vi "UpdateWeeks (SubVI).vi"(8 "Error In":errorcluster, 11 "DVR In":refnum<data-value>) -> (0 "Error Out":errorcluster, 1 "End Date":timestamp, 2 "Start Date":timestamp, 3 "DVR Out":refnum<data-value>)   [LabVIEW 2017, in "DS_Lib.lvlib" / "SRReportParser.lvlib"]
uses:
  SRReportParser.lvlib
  Modules/Private Controls/Report Data Cluster.ctl
  Modules/Private Controls/Data Raw.ctl
  Modules/Data Operations.lvlib
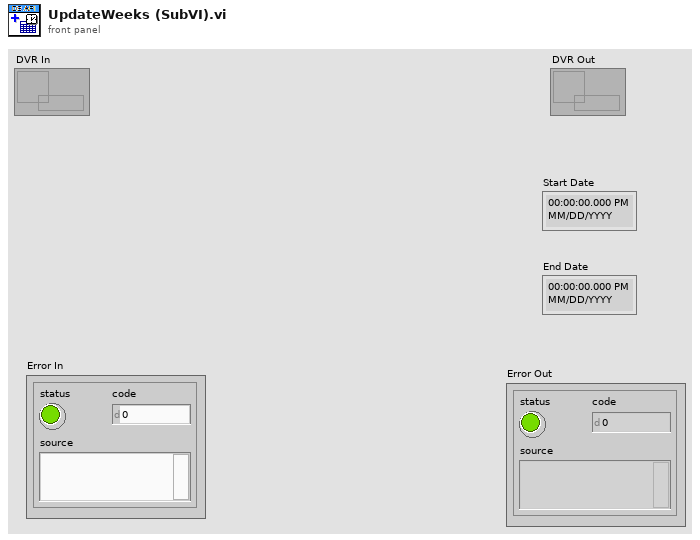
[diagram p1: front panel]
types:
  T1 = typedef "Data Operations.lvlib/Report Data Cluster.ctl" = cluster{"Headers":cluster{"Start Date":timestamp, "End Date":timestamp, "SR Status String":string[], "AE Owner String":string[]}, "Data":T2[]}
  T2 = typedef "Data Operations.lvlib/Data Raw.ctl" = cluster{"SR Number":string, "Status":string, "Summary":string, "AE Owner":string, "AE Group":string, "Contact":string, "SurveyData":cluster{"Resolution Time":dbl, "Total Satisfaction":dbl, "Response Time":dbl, "Courtesy":dbl, "Problem Solved":dbl, "Level of effort":dbl}, "Time Data":cluster{"Last Update Date":timestamp, "Creation Date":timestamp, "Creation week":i16, "Last Update Week":i16, "Creation Year":i16}}
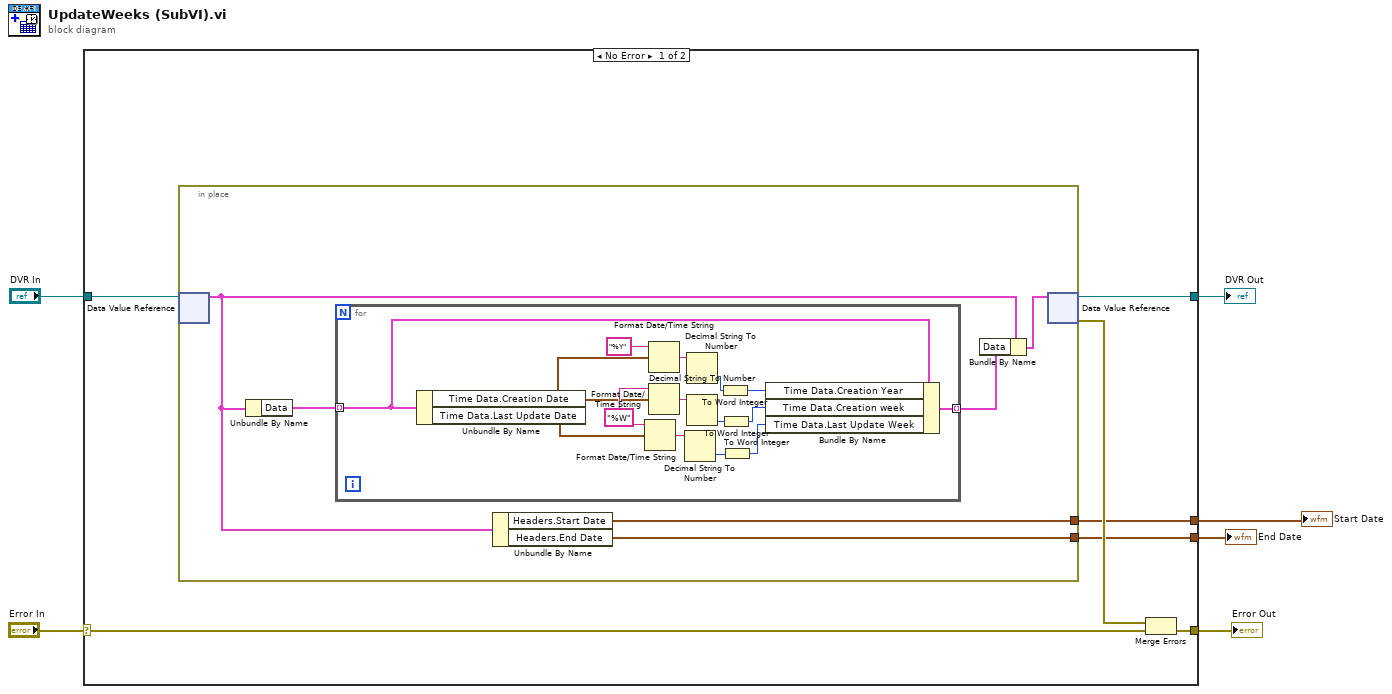
[diagram p0: block diagram]
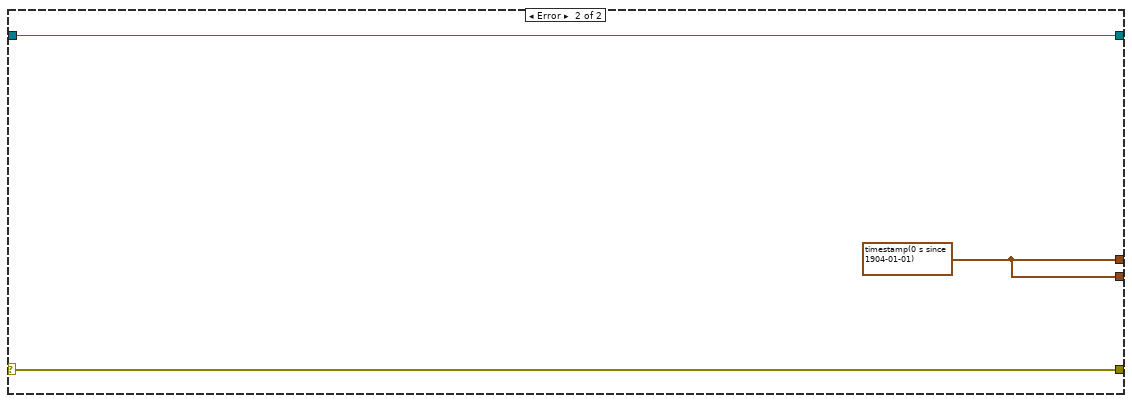
[diagram p2: hidden frame]
diagram:
  n1 = case shown="No Error" "Error In" {
    selector: "Error In" -> [w12 w37]
    tunnel: [w11 w37] -> w5
    tunnel: "DVR In" -> [w10 w36]
    tunnel: [w9 w36] -> w3
    tunnel: [w8 w35] -> w2
    tunnel: [w7 w35] -> w1
    frame No Error {
      n2 = in-place {
        in-place-border: [w15] -> w8
        in-place-border: [w14] -> w7
        n3 = in-place-dvr #1(w10) -> (w16:T1)  [unwired: 1 out]
        n4 = Unbundle By Name(w16) -> ("Data"=w19:T2[])
        n5 = for {
          tunnel: w19 -> [w34] mode=indexing
          tunnel: [w32] -> w18 mode=indexing
          w29 = "%W" ("time format string (%c)")
          n6 = Unbundle By Name(w34) -> ("Time Data.Creation Date"=w26:timestamp, "Time Data.Last Update Date"=w30:timestamp)
          n7 = Format Date/Time String(time format string (%c)=w29, seconds (now)=w30) -> (date/time string=w31:string)  [unwired: 1 in]
          n8 = Format Date/Time String(time format string (%c)="%Y", seconds (now)=w26) -> (date/time string=w28:string)  [unwired: 1 in]
          n9 = Format Date/Time String(time format string (%c)=w29, seconds (now)=w26) -> (date/time string=w33:string)  [unwired: 1 in]
          n10 = Decimal String To Number(string=w31) -> (number=w24:i32)  [unwired: 2 in, 1 out]
          n11 = Decimal String To Number(string=w28) -> (number=w25:i32)  [unwired: 2 in, 1 out]
          n12 = Decimal String To Number(string=w33) -> (number=w23:i32)  [unwired: 2 in, 1 out]
          n13 = To Word Integer(number=w25) -> (16bit integer=w20:i16)
          n14 = To Word Integer(number=w23) -> (16bit integer=w22:i16)
          n15 = To Word Integer(number=w24) -> (16bit integer=w21:i16)
          n16 = Bundle By Name(cluster=w34, "Time Data.Creation Year"=w20, "Time Data.Creation week"=w22, "Time Data.Last Update Week"=w21) -> (w32:T2)
        }
        n17 = Unbundle By Name(w16) -> ("Headers.Start Date"=w14:timestamp, "Headers.End Date"=w15:timestamp)
        n18 = Bundle By Name(cluster=w16, "Data"=w18) -> (w17:T1)
        n19 = in-place-dvr #1(w17) -> (w9:refnum<data-value>, w13:errorcluster)
      }
      n20 = Merge Errors(w13, w12) -> (w11:errorcluster)
    }
    frame Error {
      w35 = timestamp(0 s since 1904-01-01) ("Start Date")
    }
  }
  "Error Out" <- w5
  "DVR Out" <- w3
  "End Date" <- w2
  "Start Date" <- w1
